vi "Object Array Pointer.vi"() -> ()   [LabVIEW 2016]
uses:
  Typedefs/Transfer Direction.ctl
  Typedefs/Block Descriptor.ctl
  Classes/Runtime/Transfer/Runtime.Transfer.lvclass
  Classes/Runtime/Channel/Runtime.Channel.lvclass
  Class 2345678.lvclass
  <vilib>/NI Veristand/VeriStand Data/Typedefs/Typedefs.Data Types.ctl
  Classes/Runtime/Channel/Runtime.Channel.lvclass/Runtime.Channel.ctl
  Classes/Runtime/Transfer/Runtime.Transfer.lvclass/Runtime.Transfer.ctl
  Classes/Runtime/Transfer/Properties/Write direction.vi
  Classes/Runtime/Transfer/Properties/Write byte order.vi
  Classes/Runtime/Channel/Properties/Write data type.vi
  Classes/Runtime/Transfer/Properties/Write Channel Runtimes.vi
  Classes/Runtime/Transfer/Properties/Read direction.vi
  Classes/Runtime/Transfer/Properties/Read byte order.vi
  Classes/Runtime/Transfer/Properties/Read Channel Runtimes.vi
  Data Sharing Framework.Configuration.lvlib
  <vilib>/NI Veristand/VeriStand Data/VeriStand Data.lvlib
  APIs/Runtime/Data Sharing Framework.Runtime.lvlib
panel:
  out "size(s)":i32
  out "*(type *) &x":i32
  out "x-y*floor(x/y)":i32
  out "size 10":i32 format="%d bytes"
  out "substring":string
  in  "offset":i32=10
  out "size 9":i32 format="%d bytes"
  out "after substring":string
  out "size 8":i32 format="%d bytes"
  out "data string 2":string
  out "unsigned byte array":u8[](array[numeric]) format="%x"
  in  "String":string
  out "data string":string
  out "size 7":i32 format="%d bytes"
  out "size 6":i32 format="%d bytes"
  out "block descriptor":T1 {"pointer" format="%016x"}
  out "size 5":i32 format="%d bytes"
  out "size 4":i32 format="%d bytes"
  out "size 3":i32 format="%d bytes"
  out "size 2":i32 format="%d bytes"
  out "channels 1":i32
  out "byte order 1":T2(ring)
  out "direction 1":T3
  out "channels 0":i32
  out "byte order 0":T2(ring)
  out "direction 0":T3
  out "size":i32 format="%d bytes"
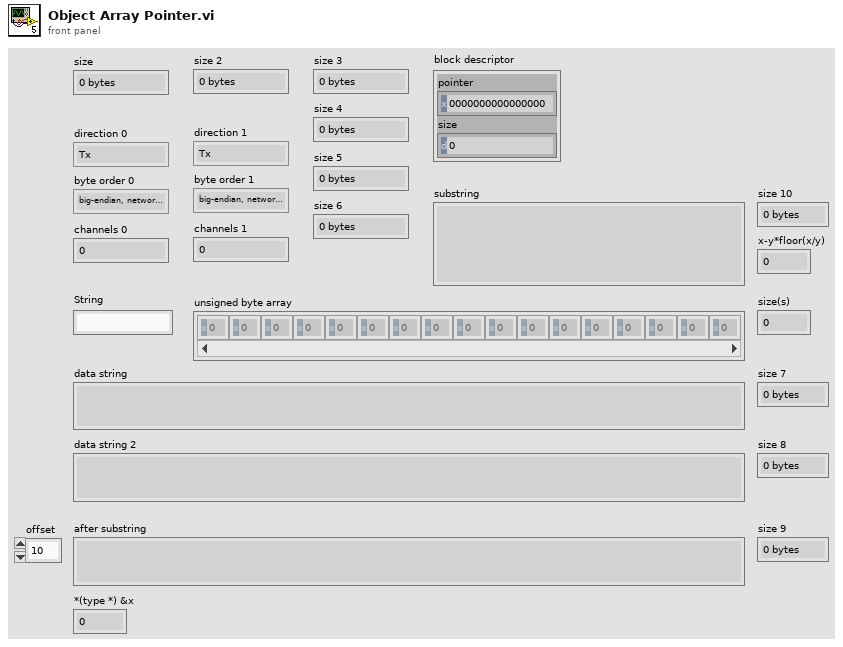
[diagram p1: front panel]
types:
  T1 = typedef "Data Sharing Framework.Runtime.lvlib/Block Descriptor.ctl" = cluster{"pointer":u64, "size":u64}
  T2 = enum16{"big-endian, network order", "native, host order", "little-endian"}
  T3 = typedef "Data Sharing Framework.Configuration.lvlib/Transfer Direction.ctl" = enum16{"Tx", "Rx"}
  T4 = typedef "VeriStand Data.lvlib/Typedefs.Data Types.ctl" = enum16{"Boolean", "Single", "Double", "I8", "I16", "I32", "I64", "U8", "U16", "U32", "U64"}
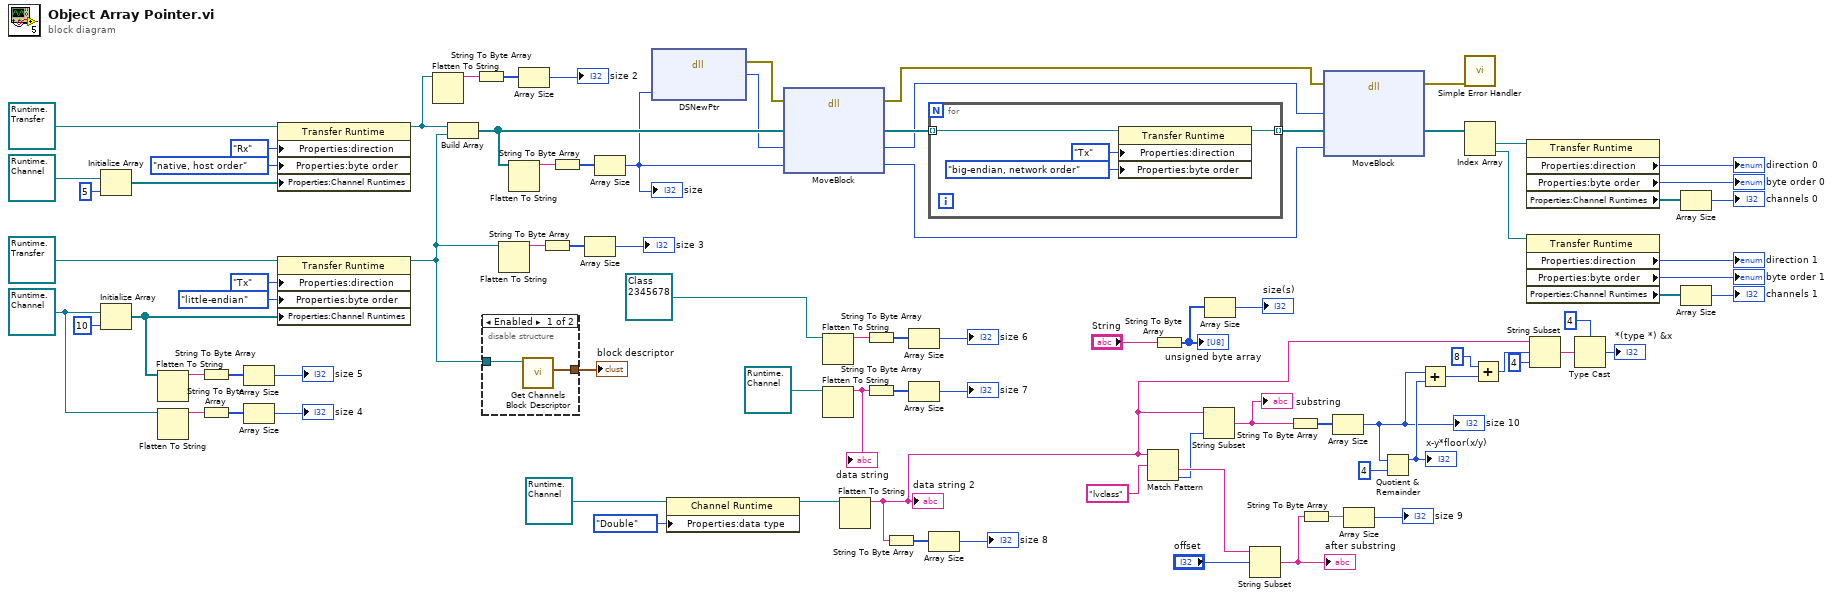
[diagram p0: block diagram]
diagram:
  w43 = refnum<class "Runtime.Channel.lvclass"> refnum ("Data Sharing Framework.Runtime.lvlib:Channel Runtime")
  n1 = Initialize Array(refnum<class "Runtime.Channel.lvclass"> refnum ("Data Sharing Framework.Runtime.lvlib:Channel Runtime"), 5 ("dimension size")) -> (w75:refnum<class "Runtime.Channel.lvclass">[])
  n2 = Initialize Array(w43, 10 ("dimension size")) -> (w39:refnum<class "Runtime.Channel.lvclass">[])
  n3 = Flatten To String(anything=w39) -> (data string=w40:string)  [unwired: 3 in, 2 out]
  n4 = Flatten To String(anything=w43) -> (data string=w46:string)  [unwired: 3 in, 2 out]
  n5 = String To Byte Array(string=w40) -> (unsigned byte array=w41:u8[])
  n6 = String To Byte Array(string=w46) -> (unsigned byte array=w45:u8[])
  n7 = Array Size(array=w41) -> (size(s)=→"size 5":i32)
  n8 = Array Size(array=w45) -> (size(s)=→"size 4":i32)
  n9 = property class="Transfer Runtime"(reference=refnum<class "Runtime.Transfer.lvclass"> refnum ("Data Sharing Framework.Runtime.lvlib:Transfer Runtime"), "Properties:direction"=Transfer_Direction."Rx" ("direction"), "Properties:byte order"=T2."native, host order" ("byte order"), "Properties:Channel Runtimes"=w75) -> (reference out=w51:refnum<class "Runtime.Transfer.lvclass">)  [unwired: 1 in, 1 out]
  n10 = property class="Transfer Runtime"(reference=refnum<class "Runtime.Transfer.lvclass"> refnum ("Data Sharing Framework.Runtime.lvlib:Transfer Runtime"), "Properties:direction"=Transfer_Direction."Tx" ("direction"), "Properties:byte order"=T2."little-endian" ("byte order"), "Properties:Channel Runtimes"=w39) -> (reference out=w38:refnum<class "Runtime.Transfer.lvclass">)  [unwired: 1 in, 1 out]
  n11 = Flatten To String(anything=w51) -> (data string=w53:string)  [unwired: 3 in, 2 out]
  n12 = Build Array(w51, w38) -> (w74:refnum<class "Runtime.Transfer.lvclass">[])
  n13 = String To Byte Array(string=w53) -> (unsigned byte array=w52:u8[])
  n14 = disable-structure shown="Enabled" {
    disable-tunnel: w38 -> [w88 _]
    disable-tunnel: [w87 _] -> w37
    frame Enabled {
      n15 = call "Get Channels Block Descriptor.vi"("Transfer Runtime in"=w88) -> ("block descriptor"=w87:T1)  [unwired: 8 in, 2 out]
    }
    frame Disabled {
    }
  }
  "block descriptor" <- w37
  n16 = Flatten To String(anything=w38) -> (data string=w47:string)  [unwired: 3 in, 2 out]
  n17 = Flatten To String(anything=w74) -> (data string=w86:string)  [unwired: 3 in, 2 out]
  n18 = Array Size(array=w52) -> (size(s)=→"size 2":i32)
  n19 = String To Byte Array(string=w47) -> (unsigned byte array=w48:u8[])
  n20 = String To Byte Array(string=w86) -> (unsigned byte array=w85:u8[])
  n21 = Array Size(array=w48) -> (size(s)=→"size 3":i32)
  n22 = Array Size(array=w85) -> (size(s)=w71:i32)
  "size" <- w71
  n23 = dll-call lib="LabVIEW" fn="DSNewPtr"("size"=w71) -> (error out=w72:errorcluster, "pointer"=w73:u64)  [unwired: 4 in, 1 out]
  n24 = property class="Channel Runtime"(reference=refnum<class "Runtime.Channel.lvclass"> refnum ("Data Sharing Framework.Runtime.lvlib:Channel Runtime"), "Properties:data type"=Typedefs.Data_Types."Double" ("data type")) -> (reference out=w28:refnum<class "Runtime.Channel.lvclass">)  [unwired: 1 in, 1 out]
  n25 = dll-call lib="LabVIEW" fn="MoveBlock"(error in=w72, "src"=w74, "dst"=w73, "size"=w71) -> (error out=w67:errorcluster, "src"=w70:refnum<class "Runtime.Transfer.lvclass">[], "dst"=w68:u64, "size"=w69:i32)  [unwired: 3 in, 1 out]
  n26 = Flatten To String(anything=refnum<class "Class 2345678.lvclass"> refnum ("Data Sharing Framework.Runtime.lvlib:Class 2.lvclass")) -> (data string=w36:string)  [unwired: 3 in, 2 out]
  n27 = Flatten To String(anything=refnum<class "Runtime.Channel.lvclass"> refnum ("Data Sharing Framework.Runtime.lvlib:Channel Runtime")) -> (data string=w25:string)  [unwired: 3 in, 2 out]
  "data string" <- w25
  n28 = Flatten To String(anything=w28) -> (data string=w10:string)  [unwired: 3 in, 2 out]
  "data string 2" <- w10
  n29 = String To Byte Array(string=w36) -> (unsigned byte array=w35:u8[])
  n30 = String To Byte Array(string=w25) -> (unsigned byte array=w32:u8[])
  n31 = String To Byte Array(string=w10) -> (unsigned byte array=w27:u8[])
  n32 = Array Size(array=w35) -> (size(s)=→"size 6":i32)
  n33 = Array Size(array=w32) -> (size(s)=→"size 7":i32)
  n34 = for {
    tunnel: w70 -> [w92] mode=indexing
    tunnel: [w89] -> w55 mode=indexing
    n35 = property class="Transfer Runtime"(reference=w92, "Properties:direction"=Transfer_Direction."Tx" ("direction"), "Properties:byte order"=T2."big-endian, network order" ("byte order")) -> (reference out=w89:refnum<class "Runtime.Transfer.lvclass">)  [unwired: 1 in, 1 out]
  }
  n36 = Array Size(array=w27) -> (size(s)=→"size 8":i32)
  n37 = Match Pattern(string=w10, regular expression="lvclass") -> (after substring=w21:string, offset past match=w18:i32)  [unwired: 1 in, 2 out]
  n38 = String To Byte Array(string="String") -> (unsigned byte array=w3:u8[])
  "unsigned byte array" <- w3
  n39 = String Subset(string=w10, length (rest)=w18) -> (substring=w16:string)  [unwired: 1 in]
  "substring" <- w16
  n40 = Array Size(array=w3) -> (size(s)=→"size(s)":i32)
  n41 = String Subset(string=w21, offset (0)="offset") -> (substring=w20:string)  [unwired: 1 in]
  "after substring" <- w20
  n42 = String To Byte Array(string=w16) -> (unsigned byte array=w17:u8[])
  n43 = String To Byte Array(string=w20) -> (unsigned byte array=w22:u8[])
  n44 = dll-call lib="LabVIEW" fn="MoveBlock"(error in=w67, "src"=w68, "dst"=w55, "size"=w69) -> (error out=w66:errorcluster, "dst"=w54:refnum<class "Runtime.Transfer.lvclass">[])  [unwired: 5 in, 1 out]
  n45 = Array Size(array=w17) -> (size(s)=w13:i32)
  "size 10" <- w13
  n46 = Array Size(array=w22) -> (size(s)=→"size 9":i32)
  n47 = Quotient & Remainder(x=w13, y=4) -> (x-y*floor(x/y)=w14:i32)  [unwired: 1 out]
  "x-y*floor(x/y)" <- w14
  n48 = Add(x=w13, y=w14) -> (x+y=w12:i32)
  n49 = call <vilib>:"Simple Error Handler.vi"("error in (no error)"=w66) -> ()  [unwired: 4 in, 5 out]
  n50 = Index Array(array=w54) -> (element #1=w57:refnum<class "Runtime.Transfer.lvclass">, element #2=w56:refnum<class "Runtime.Transfer.lvclass">)  [unwired: 2 in]
  n51 = Add(x=8, y=w12) -> (x+y=w9:i32)
  n52 = property class="Transfer Runtime"(reference=w57) -> ("Properties:direction"=→"direction 0":T3, "Properties:byte order"=→"byte order 0":T2, "Properties:Channel Runtimes"=w65:refnum<class "Runtime.Channel.lvclass">[])  [unwired: 1 in, 2 out]
  n53 = property class="Transfer Runtime"(reference=w56) -> ("Properties:direction"=→"direction 1":T3, "Properties:byte order"=→"byte order 1":T2, "Properties:Channel Runtimes"=w61:refnum<class "Runtime.Channel.lvclass">[])  [unwired: 1 in, 2 out]
  n54 = String Subset(string=w10, offset (0)=w9, length (rest)=4 ("length (rest)")) -> (substring=w7:string)
  n55 = Type Cast(type=4 ("length (rest)"), x=w7) -> (*(type *) &x=→"*(type *) &x":i32)
  n56 = Array Size(array=w65) -> (size(s)=→"channels 0":i32)
  n57 = Array Size(array=w61) -> (size(s)=→"channels 1":i32)
